vi "root Folder.vi"() -> (3 "root folder":path)   [LabVIEW 2019, in "SLMP.lvlib"]
uses:
  SLMP.lvlib
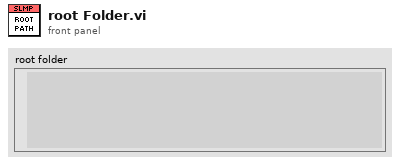
[diagram p1: front panel]
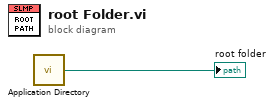
[diagram p0: block diagram]
diagram:
  n1 = call <vilib>:"Application Directory.vi"() -> ("Application Directory"=→"root folder":path)
